vi "batch processor.vi"() -> ()   [LabVIEW 2013]
uses:
  <vilib>/Utility/miscctls.llb/LVPointTypeDef.ctl
  <userlib>/Accelerator/User Interface/Controls/Post_Dust_Event.ctl
  <userlib>/Accelerator/User Interface/Controls/File_location.ctl
  <userlib>/Accelerator/User Interface/Controls/Post_Dust_Event_small.ctl
  <userlib>/_OpenG.lib/array/array.llb/Slice 1D Array (DBL)__ogtk.vi
  <userlib>/Accelerator/Sub-Polymorphic/update_dust_event_big.vi
  <userlib>/_OpenG.lib/string/string.llb/Trim Whitespace (String)__ogtk.vi
  <userlib>/Accelerator/Sub-Polymorphic/update_dust_event_small.vi
  <userlib>/_OpenG.lib/array/array.llb/Empty 1D Array (String)__ogtk.vi
  <vilib>/addons/database/_DB Variant To Data/Database Variant To Data.xnode
panel:
  out "All Processing Frequencies":dbl[](array[numeric])
  in  "Live Run?":bool
  out "Last live data":timestamp
  out "Timed out?":bool
  in  "Tab Control":T1(tab)
  out "Small?":bool
  in  "Clear IDL Errors":bool
  out "IDL Errors":errorcluster
  out "Test":bool caption="Test Database in use:"
  out "Production":bool=TRUE caption="Production Database in use:"
  out "Events being processed:":i32
  out "Processing Frequency (Hz):":ext=3.0
  out "Database Update Progress:":u8(slide) scale=0.0..100.0
  out "IDL Code Executing":bool=TRUE
  out "Estimated IDL Progress:":u8(slide) scale=0.0..100.0
  out "standard error":string
  out "standard output":string
  out "Processing Old Data":bool
  out "Estimated processing time":string="0 days, 0 h, 0 m, 0 s."
  out "Estimated end time":timestamp format="%<%X\n%x>T"
  out "Quality":ext format="%.2f"
  out "Charge":ext
  out "Velocity":ext
  out "Time taken by IDL per shot: (s)":dbl=0.25
  out "Shot being processed:":string
  out "Remaining Shots:":string
  out "Output to IDL command line:":string="\"C:\\Program Files\\Exelis\\IDL82\\bin\\bin.x86_64\\idl.exe\" -e  \"idl_batch_processor, 'X:'\""
  out "Estimate time to process":string="0 s."
  out "Estimate stop time":timestamp format="%<%X\n%x>T"
  out "Total Events":i64
  in  "Lower Time Stamp":timestamp
  in  "Upper Time Stamp":timestamp
  in  "Process old data":bool
  in  "Search Times":bool
  in  "Process all errored entries":bool
  in  "stop":bool
  # "Database Update System V2"
  # "You can ALWAYS run the accelerator.\n\nThis will continue to update the Live\nPlot even if it is processing old data."
  # "Error Status:"
  # "ODBC Connection Status:"
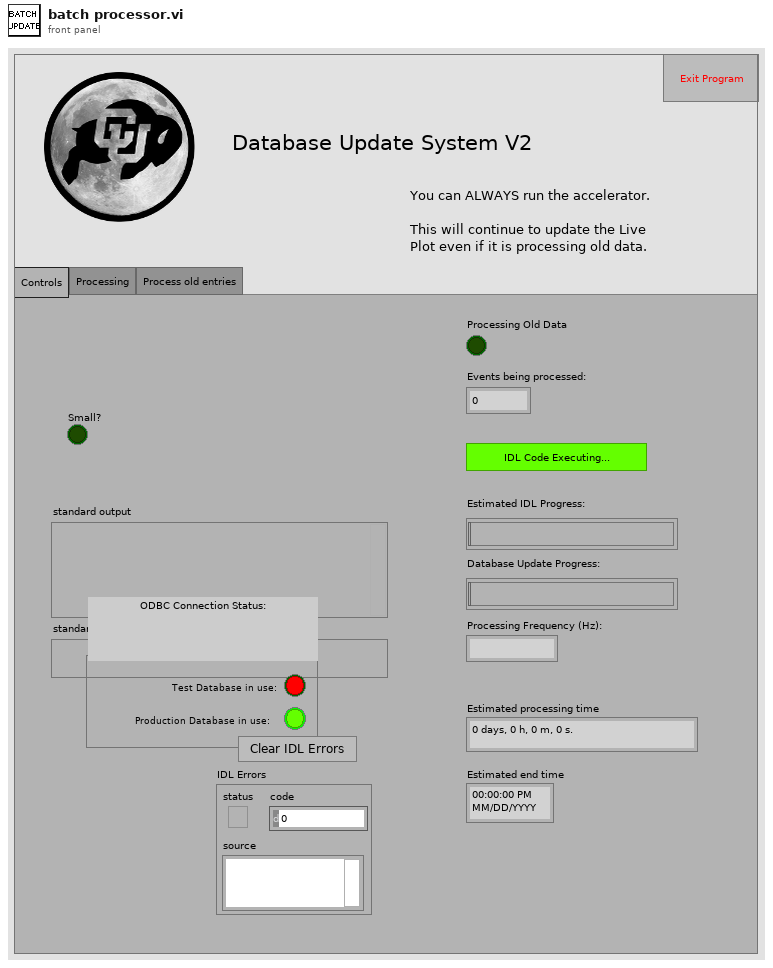
[diagram p1: front panel]
types:
  T1 = enum32{"Controls", "Processing", "Process old entries"}
  T2 = typedef "LVPointTypeDef.ctl" = cluster{"Horizontal":i16, "Vertical":i16}
  T3 = enum8{"Enabled", "Disabled", "Disabled and Grayed Out"}
  T4 = enum16{"open", "replace", "create", "open or create", "replace or create", "replace or create with confirmation"}
  T5 = typedef "Post_Dust_Event.ctl" = cluster{"Dust Event ID":i64, "Integer Timestamp":i64, "Velocity":sgl, "Mass":sgl, "Charge":sgl, "Radius":sgl, "Experiment Settings":dbl, "Pelletron ID":i32, "Estimate Quality":sgl, "File Location":T6, "id_dust_info":dbl, "DCS 1 X":sgl, "DCS 1 Y":sgl, "DCS 2 X":sgl, "DCS 2 Y":sgl}
  T6 = typedef "File_location.ctl" = i8
  T7 = typedef "Post_Dust_Event_small.ctl" = cluster{"Dust Event ID":i64, "Integer Timestamp":i64, "Velocity":sgl, "Mass":sgl, "Charge":sgl, "Radius":sgl, "Needle Voltage (MV)":dbl, "Experiment Settings":dbl, "Estimate Quality":sgl, "File Location":T6, "id_dust_info":dbl}
  T8 = typedef "bp_cluster.ctl" = cluster{"Dust Event ID":i64, "High Voltage":sgl, "Experiment Settings  ID":i64, "File Location":T6, "Dust Density":dbl}
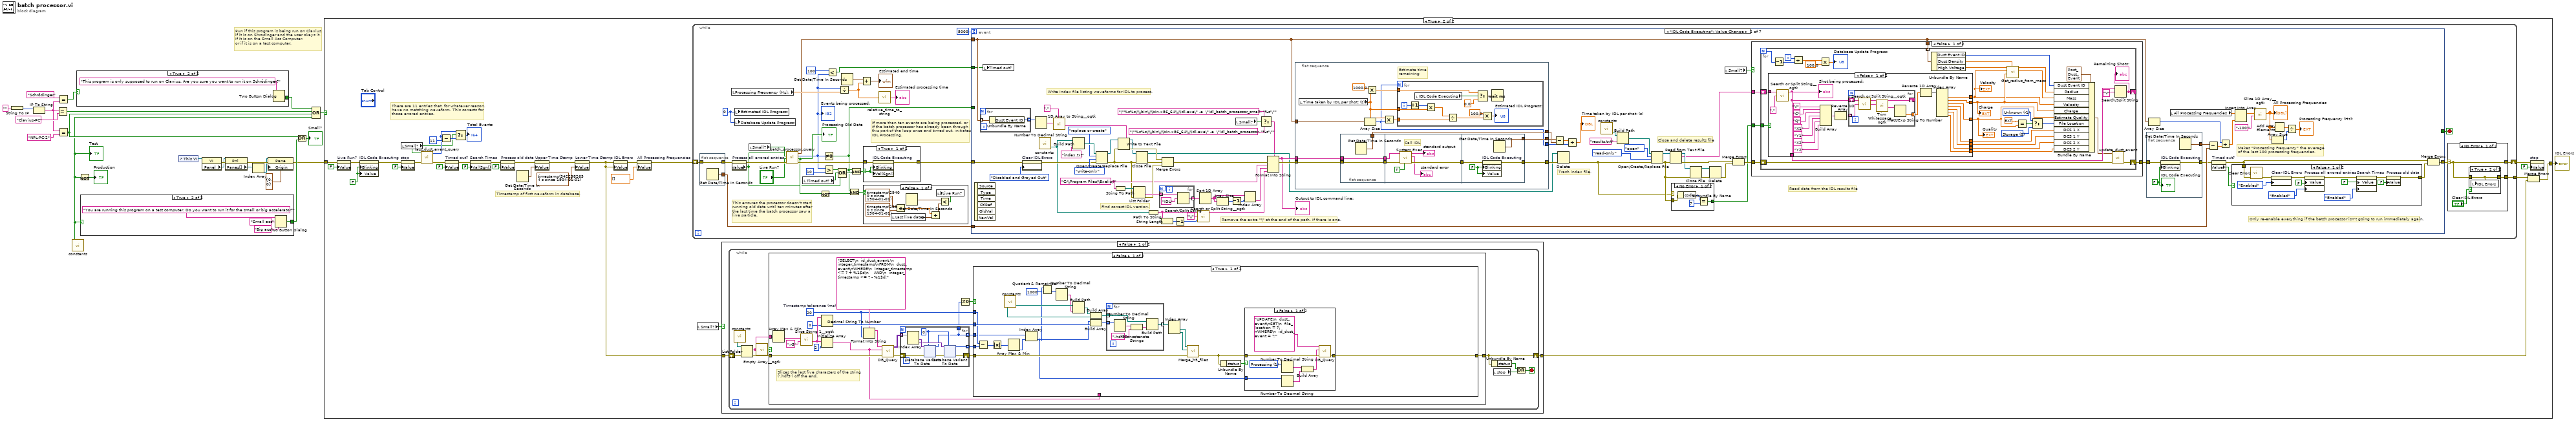
[diagram p0: block diagram]
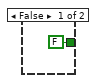
[diagram p2: hidden frame]
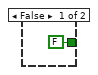
[diagram p3: hidden frame]
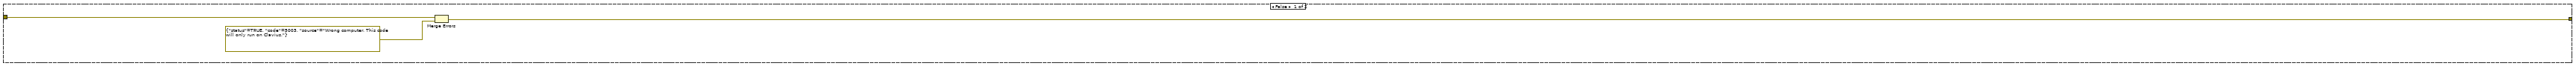
[diagram p4: hidden frame]
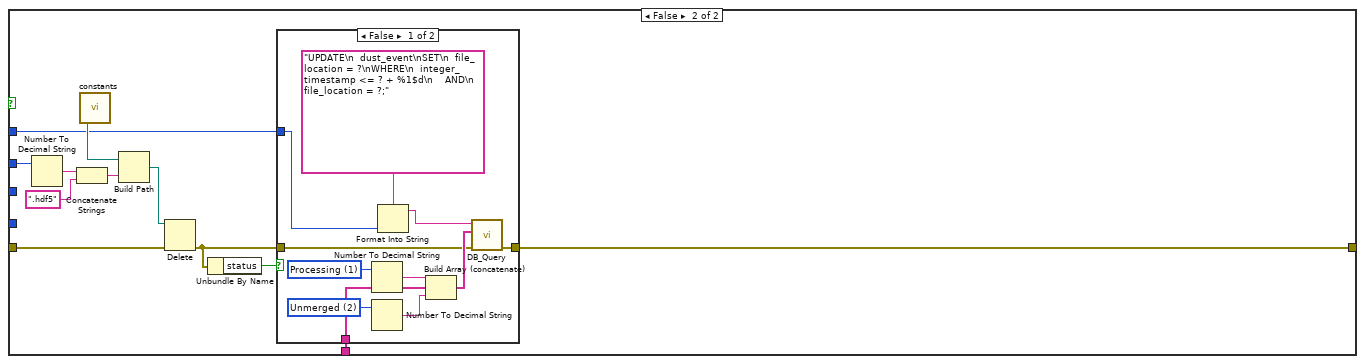
[diagram p6: hidden frame]
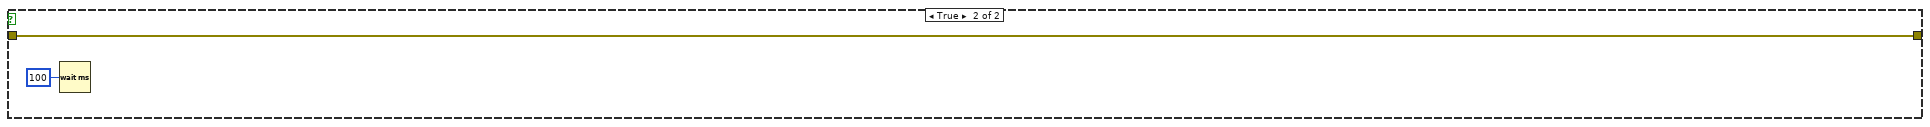
[diagram p8: hidden frame]
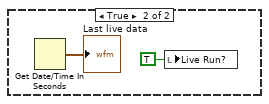
[diagram p10: hidden frame]
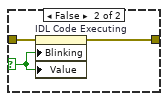
[diagram p11: hidden frame]
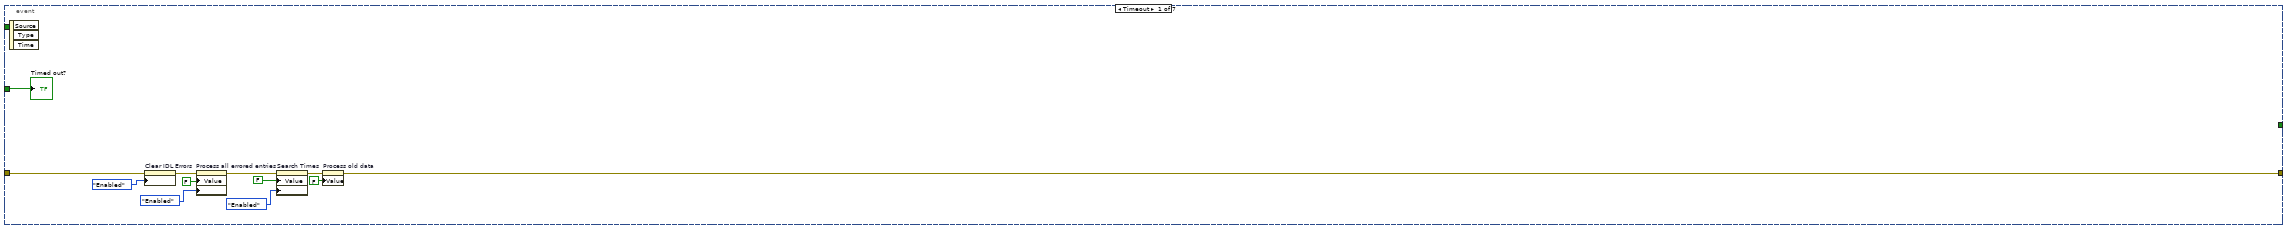
[diagram p12: hidden frame]
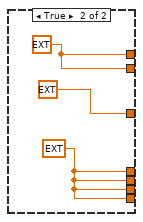
[diagram p13: hidden frame]
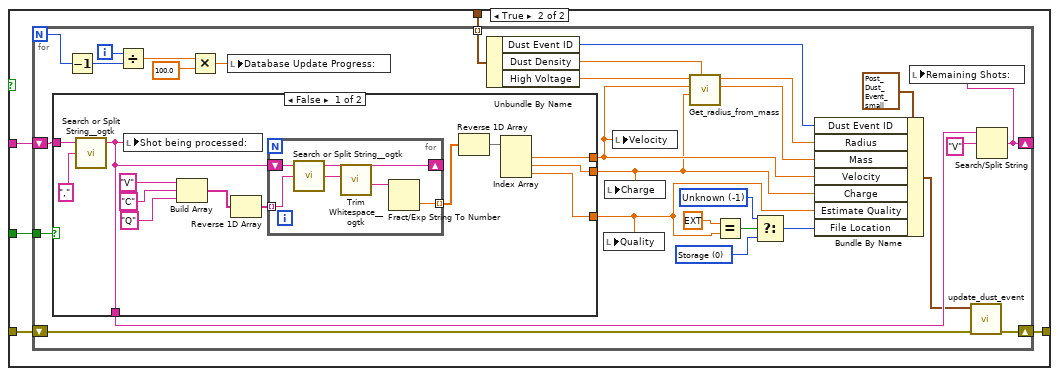
[diagram p14: hidden frame]
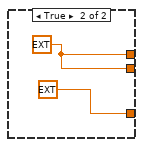
[diagram p15: hidden frame]
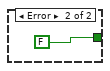
[diagram p17: hidden frame]
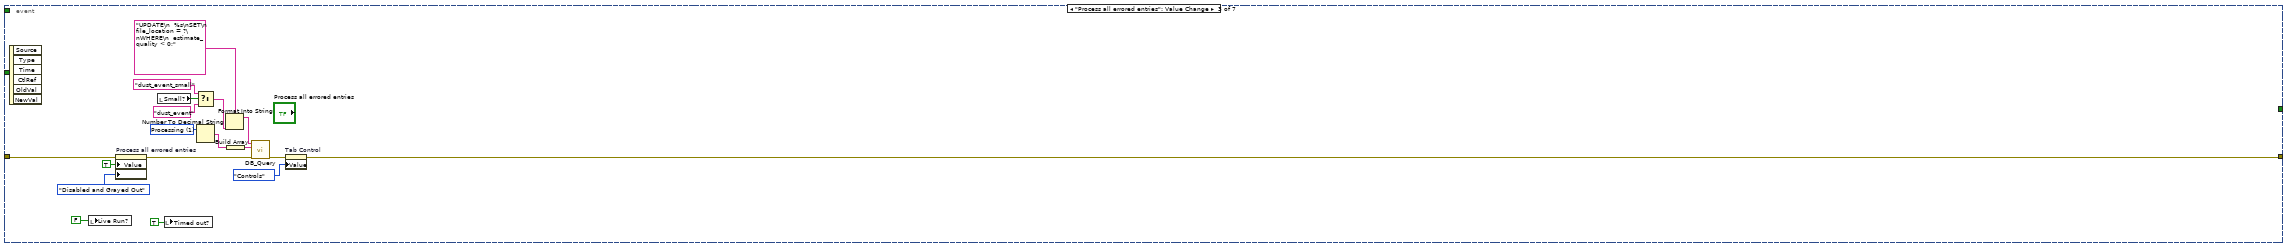
[diagram p18: hidden frame]
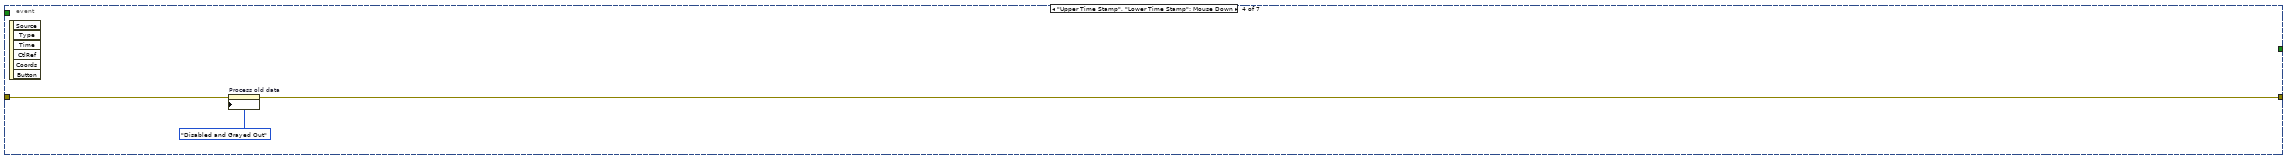
[diagram p19: hidden frame]
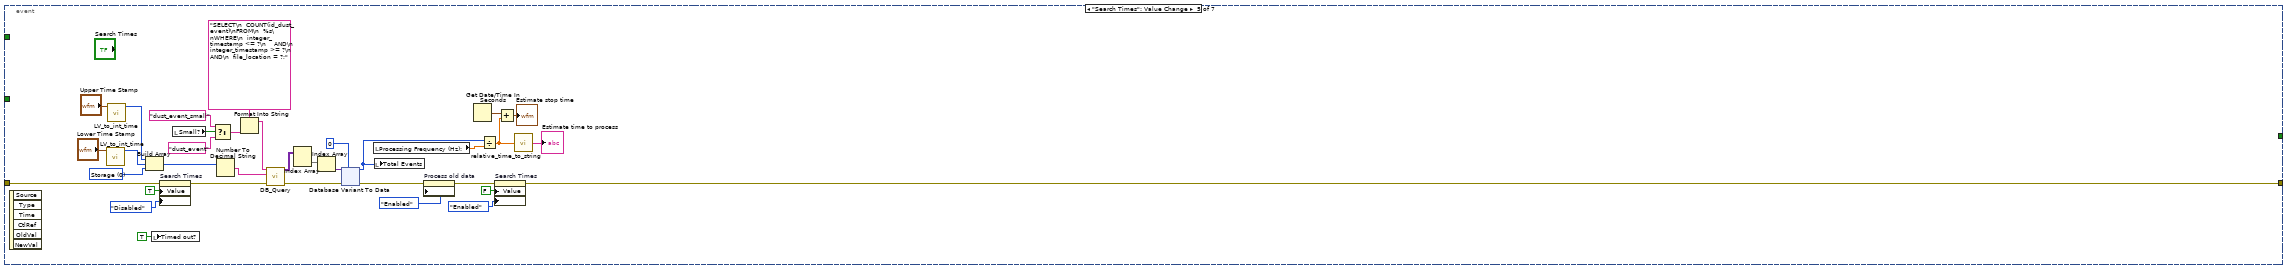
[diagram p20: hidden frame]
diagram:
  # "Run if this program is being run on Clavius,\nif it is on Shrodinger and the user okays it,\nif it is on the Small Acc Computer,\nor if it is on a test computer."
  n1 = String To IP(1:"" ("name")) -> (0:w17:u32)
  n2 = IP To String(2:w17) -> (0:w7:string)  [unwired: 1 in]
  n3 = Equal?(x=w7, y="Clavius-PC") -> (x = y?=w12:bool)
  n4 = Equal?(x="Schrödinger", y=w7) -> (x = y?=w10:bool)
  n5 = Equal?(x=w7, y="NPL-PC-2") -> (x = y?=w5:bool)
  n6 = call <userlib>:"constants.vi"() -> ("Testing"=w1:bool)  [unwired: 3 out]
  "Test" <- w1
  n7 = case shown="True" w10 {
    tunnel: [FALSE ("T button?") w27] -> w11
    frame False {
    }
    frame True {
      n8 = Two Button Dialog(message="This program is only supposed to run on Clavius. Are you sure you want to run it on Schrödinger?") -> (T button?=w27:bool)  [unwired: 2 in]
    }
  }
  n9 = Not(x=w1) -> (.not. x?=→"Production":bool)
  n10 = case shown="True" w1 {
    tunnel: [FALSE ("T button?") w32] -> w4
    frame False {
    }
    frame True {
      n11 = Two Button Dialog(message="You are running this program on a test computer. Do you want to run it for the small or big accelerator?", 1:"Big acc" ("F button name (\"Cancel\")"), 2:"Small acc" ("T button name (\"OK\")")) -> (T button?=w32:bool)
    }
  }
  n12 = control-ref of="This VI"() -> (w24:refnum<vi>)
  n13 = property class="VI"(reference=w24) -> (error out=w23:errorcluster, "Panel"=w22:refnum<vi>)  [unwired: 1 in, 1 out]
  n14 = property class="Pnl"(reference=w22, error in=w23) -> (error out=w21:errorcluster, "Panes[]"=w20:refnum<vi>[])  [unwired: 1 out]
  n15 = Index Array(array=w20) -> (element=w19:refnum<vi>)  [unwired: 1 in]
  n16 = property class="Pane"(reference=w19, error in=w21, "Origin"=T2 {"Horizontal"=0, "Vertical"=0}) -> (error out=w3:errorcluster)  [unwired: 1 out]
  n17 = Or(x=w5, y=w4) -> (x .or. y?=→"Small?":bool)
  n18 = Compound Arithmetic op=OR(w11, w12, w5, w1) -> (w9:bool)
  n19 = case shown="True" w9 {
    tunnel: w3 -> [w35 w41]
    tunnel: [w33 w37] -> w14
    frame False {
      n20 = Merge Errors(w35, errorcluster {"status"=TRUE, "code"=5003, "source"="Wrong computer. This code will only run on Clavius."} ("error IO")) -> (w33:errorcluster)
    }
    frame True {
      w67 = FALSE ("IDL Code Executing")
      # "There are 11 entries that, for whatever reason,\nhave no matching waveform. This corrects for\nthose errored entries."
      # "Timestamp of first waveform in database."
      n21 = property on="Live Run?" class="Bool (strict)"(error in=w41, "Value"=FALSE ("Live Run?")) -> (error out=w50:errorcluster)  [unwired: 1 in, 1 out]
      n22 = property on="IDL Code Executing" class="Bool (strict)"(error in=w50, "Blinking"=w67, "Value"=w67) -> (error out=w64:errorcluster)  [unwired: 1 in, 1 out]
      n23 = property on="stop" class="Bool (strict)"(error in=w64, "Value"=FALSE ("stop")) -> (error out=w54:errorcluster)  [unwired: 1 in, 1 out]
      n24 = local read "Small?"() -> (w42:bool)
      n25 = call <userlib>:"last_dust_event_query.vi"("error in (no error)"=w54, "Small?"=w42) -> ("error out"=w53:errorcluster, "id_dust_event"=w43:i64)  [unwired: 8 in]
      n26 = Subtract(x=w43, y=i64 11) -> (x-y=w44:i64)
      n27 = property on="Timed out?" class="Bool (strict)"(error in=w53, "Value"=FALSE ("stop")) -> (error out=w58:errorcluster)  [unwired: 1 in, 1 out]
      n28 = Select(t=w43, s=w42, f=w44) -> (s? t:f=→"Total Events":i64)
      n29 = property on="Search Times" class="Bool (strict)"(error in=w58, "Val(Sgnl)"=FALSE ("Search Times")) -> (error out=w56:errorcluster)  [unwired: 1 in, 1 out]
      n30 = property on="Process old data" class="Bool (strict)"(error in=w56, "Value"=FALSE ("Process old data")) -> (error out=w51:errorcluster)  [unwired: 1 in, 1 out]
      n31 = Get Date/Time In Seconds() -> (seconds since 1Jan1904=w62:timestamp)
      n32 = property on="Upper Time Stamp" class="AbsTime (strict)"(error in=w51, "Value"=w62) -> (error out=w61:errorcluster)  [unwired: 1 in, 1 out]
      n33 = property on="Lower Time Stamp" class="AbsTime (strict)"(error in=w61, "Value"=timestamp(3422982654.564 s since 1904-01-01) ("Upper Time Stamp")) -> (error out=w40:errorcluster)  [unwired: 1 in, 1 out]
      n34 = property on="IDL Errors" class="Clust (strict)"(error in=w40, "Value"=w40) -> (error out=w48:errorcluster)  [unwired: 1 in, 1 out]
      n35 = property on="All Processing Frequencies" class="Arr (strict)"(error in=w48, "Value"=dbl[] [] ("All Processing Frequencies")) -> (error out=w46:errorcluster)  [unwired: 1 in, 1 out]
      n36 = while {
        shift-right: [w265] -> w65
        shift-left: w46 -> [w254]
        tunnel: [w264] -> w38
        stop <- w260 stop-if-true
        w268 = u8 0 ("Database Update Progress")
        # "This ensures the processor doesn't start\nrunning old data until ten minutes after\nthe last time the batch processor saw a\nlive particle."
        # "If more than ten events are being processed, or\nif the batch processor has already been through\nthis part of the loop once and timed out, initiates\nIDL Processing."
        n37 = flat-sequence {
          tunnel: [w279] -> w255
          tunnel: w254 -> [w279]
          tunnel: [w278] -> w253
          frame #0 {
            n38 = Get Date/Time In Seconds() -> (seconds since 1Jan1904=w278:timestamp)
          }
        }
        n39 = local read "Processing Frequency (Hz):"() -> (w245:ext)
        n40 = property on="Process all errored entries" class="Bool (strict)"(error in=w255) -> (error out=w259:errorcluster, "Value"=w241:bool)  [unwired: 1 in, 1 out]
        n41 = local write "Estimated IDL Progress:"(w268) -> ()
        n42 = local write "Database Update Progress:"(w268) -> ()
        n43 = local read "Small?"() -> (w252:bool)
        n44 = call <userlib>:"batch_processor_query.vi"("error in (no error)"=w259, "Live Run?"="Live Run?", "Small?"=w252, "Update Error files?"=w241) -> ("error out"=w262:errorcluster, "Old Processing"=w248:bool, "Total Events"=w237:i32, "BP Array"=w236:T8[])  [unwired: 4 in]
        "Events being processed:" <- w237
        "Processing Old Data" <- w248
        n45 = local read "Timed out?"() -> (w256:bool)
        n46 = Not(x=w248) -> (.not. x?=w247:bool)
        n47 = Not Equal To 0?(x=w237) -> (x != 0?=w240:bool)
        n48 = Greater?(x=w237, y=10) -> (0:w258:bool)
        n49 = Less?(x=100 ("length"), y=w237) -> (x < y?=w238:bool)
        n50 = Compound Arithmetic op=OR(w258, w256, w241) -> (w251:bool)
        n51 = Divide(x=w237, y=w245) -> (x/y=w243:ext)
        n52 = Get Date/Time In Seconds() -> (seconds since 1Jan1904=w246:timestamp)
        n53 = And(x=w240, y=w247) -> (x .and. y?=w249:bool)
        n54 = And(x=w240, y=w251) -> (x .and. y?=w257:bool)
        n55 = Add(x=w246, y=w243) -> (x+y=→"Estimated end time":timestamp)
        n56 = case shown="True" w257 {
          selector: w257 -> [w280 w283]
          tunnel: w262 -> [w282 w285]
          tunnel: [w281 w284] -> w261
          frame True {
            n57 = property on="IDL Code Executing" class="Bool (strict)"(error in=w282, "Blinking"=w280, "Val(Sgnl)"=w280) -> (error out=w281:errorcluster)  [unwired: 1 in, 1 out]
          }
          frame False {
            n58 = property on="IDL Code Executing" class="Bool (strict)"(error in=w285, "Blinking"=w283, "Value"=w283) -> (error out=w284:errorcluster)  [unwired: 1 in, 1 out]
          }
        }
        n59 = case shown="False" w249 {
          frame False {
            n60 = local read "Last live data"() -> (w275:timestamp)
            n61 = Subtract(x=timestamp(29400 s since 1904-01-01) ("Last live data"), y=timestamp(28800 s since 1904-01-01) ("Last live data")) -> (x-y=w274:dbl)
            n62 = Get Date/Time In Seconds() -> (seconds since 1Jan1904=w270:timestamp)
            n63 = Add(x=w274, y=w275) -> (x+y=w269:timestamp)
            n64 = Less?(x=w270, y=w269) -> (x < y?=w271:bool)
            n65 = local write "Live Run?"(w271) -> ()
          }
          frame True {
            n66 = Get Date/Time In Seconds() -> (seconds since 1Jan1904=→"Last live data":timestamp)
            n67 = local write "Live Run?"(TRUE ("Live Run?")) -> ()
          }
        }
        n68 = call <userlib>:"relative_time_to_string.vi"("Seconds"=w243) -> ("String time"=→"Estimated processing time":string)
        n69 = event shown="[1] \"IDL Code Executing\": Value Change" {
          selector: _ -> [_ _ _ _ _ _ _]
          dyn-events: _ -> [_ _ _ _ _ _ _]
          timeout: 5000 -> [_ _ _ _ _ _ _]
          tunnel: w261 -> [w288 w325 w582 w588 w604 w663 w683]
          tunnel: w236 -> [_ w315 _ _ _ _ _]
          tunnel: [w287 w322 w586 w587 w612 w677 w683] -> w266
          tunnel: [_ _ _ _ _ _ "stop"] -> w260
          tunnel: w253 -> [_ w316 _ _ _ _ _]
          tunnel: w240 -> [w286 _ _ _ _ _ _]
          tunnel: w238 -> [_ w313 _ _ _ _ _]
          event Timeout {
            n70 = event-data() -> ()  [unwired: 1 in, 3 out]
            n71 = property on="Clear IDL Errors" class="Bool"(error in=w288, "DisabledEnum"=T3."Enabled" ("Disabled")) -> (error out=w294:errorcluster)  [unwired: 1 in, 1 out]
            n72 = property on="Process all errored entries" class="Bool (strict)"(error in=w294, "Value"=FALSE ("Process old errored entries"), "DisabledEnum"=T3."Enabled" ("Disabled")) -> (error out=w295:errorcluster)  [unwired: 1 in, 1 out]
            n73 = property on="Search Times" class="Bool (strict)"(error in=w295, "Value"=FALSE ("Process old data"), "DisabledEnum"=T3."Enabled" ("Disabled")) -> (error out=w296:errorcluster)  [unwired: 1 in, 1 out]
            n74 = property on="Process old data" class="Bool (strict)"(error in=w296, "Value"=FALSE ("Process old data")) -> (error out=w287:errorcluster)  [unwired: 1 in, 1 out]
            "Timed out?" <- w286
          }
          event "IDL Code Executing": Value Change {
            w347 = "C:\\Program Files\\Exelis\\"
            # "Makes \"Processing Frequency\" the average\nof the last 100 processing frequencies."
            # "Only re-enable everything if the batch processor isn't going to run immediately again."
            # "Close and delete results file"
            # "Read data from the IDL results file"
            # "Trash index file."
            # "Remove the extra \"\\\" at the end of the path, if there is one."
            # "Find correct IDL version."
            # "Write index file listing waveforms for IDL to process."
            n75 = event-data() -> ()  [unwired: 1 in, 6 out]
            n76 = for {
              tunnel: w315 -> [w517] mode=indexing
              tunnel: [w516] -> w344 mode=indexing
              n77 = Unbundle By Name(w517) -> ("Dust Event ID"=w516:i64)
            }
            n78 = local write "Timed out?"(w313) -> ()
            n79 = property on="Clear IDL Errors" class="Bool"(error in=w325, "DisabledEnum"=T3."Disabled and Grayed Out" ("Disabled")) -> (error out=w301:errorcluster)  [unwired: 1 in, 1 out]
            n80 = Number To Decimal String(number=w344) -> (decimal integer string=w340:string[])  [unwired: 1 in]
            n81 = call <userlib>:"constants.vi"() -> ("Processed HDF5 filepath"=w300:path)  [unwired: 3 out]
            n82 = call <userlib>:"1D Array to String__ogtk.vi"("delimiter (Tab)"=",", "Array of Strings"=w340) -> ("delimited string"=w338:string)  [unwired: 9 in]
            n83 = Build Path(base path=w300, name or relative path="index.txt") -> (appended path=w378:path)
            n84 = Open/Create/Replace File(file path (use dialog)=w378, error in=w301, operation (0:open)=T4."replace or create", access (0:read/write)=enum16{"read/write", "read-only", "write-only"}."write-only") -> (refnum out=w341:refnum<file>, error out=w337:errorcluster)  [unwired: 2 in, 1 out]
            n85 = String To Path(string=w347) -> (path=w359:path)
            n86 = Write to Text File(file (use dialog)=w341, text=w338, error in=w337) -> (refnum out=w342:refnum<file>, error out=w343:errorcluster)  [unwired: 1 in, 1 out]
            n87 = List Folder(path=w359, error in=w337) -> (folder names=w358:string[], error out=w348:errorcluster)  [unwired: 2 in, 2 out]
            n88 = Close File(refnum=w342, error in=w337) -> (path=w330:path, error out=w377:errorcluster)
            n89 = Path To String(path=w300) -> (string=w350:string)
            n90 = for {
              tunnel: w358 -> [w519] mode=indexing
              tunnel: [w518] -> w356 mode=indexing
              n91 = Search/Split String(string=w519, search string/char (-)="IDL" ("Element Data")) -> (match + rest of string=w518:string)  [unwired: 1 in, 2 out]
            }
            n92 = String Length(string=w350) -> (length=w352:i32)
            n93 = Merge Errors(w343, w377, w348) -> (w370:errorcluster)
            n94 = Decrement(x=w352) -> (x-1=w351:i32)
            n95 = call <userlib>:"Search or Split String__ogtk.vi"("offset (0)"=w351, "search string/char (-)"="\\", "string"=w350) -> ("substring before match"=w345:string)  [unwired: 2 out]
            n96 = Sort 1D Array(array=w356) -> (sorted array=w357:string[])
            n97 = Array Size(array=w357) -> (size(s)=w355:i32)
            n98 = Decrement(x=w355) -> (x-1=w354:i32)
            n99 = local read "Small?"() -> (w320:bool)
            n100 = Index Array(array=w357, index=w354) -> (element=w346:string)
            n101 = Select(t="\"%s%s\\\\bin\\\\bin.x86_64\\\\idl.exe\" -e  \"idl_batch_processor_small, '%s'\"" ("format string"), s=w320, f="\"%s%s\\\\bin\\\\bin.x86_64\\\\idl.exe\" -e  \"idl_batch_processor, '%s'\"" ("format string")) -> (s? t:f=w317:string)
            n102 = Format Into String(format string=w317, error in=w370, w347, w346, w345) -> (resulting string=w353:string, error out=w371:errorcluster)  [unwired: 1 in]
            "Output to IDL command line:" <- w353
            n103 = flat-sequence {
              tunnel: w371 -> [w542]
              tunnel: w353 -> [w543]
              tunnel: [w541] -> w331
              tunnel: [w534] -> w336
              tunnel: [w533] -> w335
              tunnel: [w531] -> w333
              tunnel: w315 -> [w530]
              frame #0 {
                # "Estimate time \nremaining"
                n104 = local read "Time taken by IDL per shot: (s)"() -> (w532:dbl)
                n105 = flat-sequence {
                  tunnel: w542 -> [w557]
                  tunnel: w543 -> [w558]
                  tunnel: [w558] -> w539
                  tunnel: [w557] -> w538
                  tunnel: [w556] -> w533
                  tunnel: [w562] -> w540
                  tunnel: w539 -> [w564]
                  tunnel: w538 -> [w563]
                  tunnel: [w568] -> w534
                  tunnel: [w565] -> w541
                  tunnel: w540 -> [w566]
                  frame #0 {
                    n106 = Get Date/Time In Seconds() -> (seconds since 1Jan1904=w556:timestamp)
                  }
                  frame #1 {
                    # "Call IDL"
                    n107 = call <vilib>:"System Exec.vi"("run minimized? (F)"=TRUE, "error in (no error)"=w563, "command line"=w564) -> ("error out"=w562:errorcluster, "standard error"=→"standard error":string, "standard output"=→"standard output":string)  [unwired: 5 in, 1 out]
                  }
                  frame #2 {
                    w567 = FALSE ("IDL Code Executing")
                    n108 = property on="IDL Code Executing" class="Bool (strict)"(error in=w566, "Blinking"=w567, "Value"=w567) -> (error out=w565:errorcluster)  [unwired: 1 in, 1 out]
                    n109 = Get Date/Time In Seconds() -> (seconds since 1Jan1904=w568:timestamp)
                  }
                }
                n110 = Array Size(array=w530) -> (size(s)=w531:i32)
                n111 = Multiply(x=sgl 1000.0 ("y"), y=w532) -> (x*y=w536:dbl)
                n112 = Multiply(x=w532, y=w531) -> (x*y=w535:dbl)
                n113 = for {
                  N: w531 -> [_]
                  tunnel: w535 -> [w551]
                  tunnel: w532 -> [w554]
                  tunnel: w536 -> [w545]
                  i -> [w555]
                  n114 = Increment(x=w555) -> (x+1=w553:i32)
                  n115 = local read "IDL Code Executing"() -> (w547:bool)
                  n116 = Multiply(x=w553, y=w554) -> (x*y=w552:dbl)
                  n117 = Divide(x=w552, y=w551) -> (x/y=w550:dbl)
                  n118 = Select(t=w545, s=w547, f=0.0) -> (s? t:f=w546:dbl)
                  n119 = Multiply(x=sgl 100.0, y=w550) -> (x*y=→"Estimated IDL Progress:":dbl)
                  n120 = Wait (ms)(milliseconds to wait=w546) -> ()  [unwired: 1 out]
                }
              }
            }
            n121 = Subtract(x=w336, y=w335) -> (x-y=w334:dbl)
            n122 = Delete(path (use dialog)=w330, error in=w331) -> (error out=w332:errorcluster)  [unwired: 3 in, 2 out]
            n123 = Divide(x=w334, y=w333) -> (x/y=→"Time taken by IDL per shot: (s)":dbl)
            n124 = call <userlib>:"constants.vi"() -> ("Processed HDF5 filepath"=w299:path)  [unwired: 3 out]
            n125 = Build Path(base path=w299, name or relative path="results.txt") -> (appended path=w375:path)
            n126 = Open/Create/Replace File(file path (use dialog)=w375, error in=w332, operation (0:open)=T4."open", access (0:read/write)=enum16{"read/write", "read-only", "write-only"}."read-only") -> (refnum out=w374:refnum<file>, error out=w361:errorcluster)  [unwired: 2 in, 1 out]
            n127 = Read from Text File(file (use dialog)=w374, error in=w361) -> (refnum out=w365:refnum<file>, text=w364:string, error out=w373:errorcluster)  [unwired: 2 in, 1 out]
            n128 = case shown="No Error" w332 {
              tunnel: w361 -> [w524 _]
              tunnel: [w521 FALSE] -> w360
              frame No Error {
                n129 = Unbundle By Name(w524) -> ("code"=w523:i32)
                n130 = Equal?(x=w523, y=7) -> (x = y?=w521:bool)
              }
              frame Error {
              }
            }
            n131 = Close File(refnum=w365, error in=w361) -> (path=w329:path, error out=w327:errorcluster)
            n132 = Delete(path (use dialog)=w329, error in=w327) -> (error out=w326:errorcluster)  [unwired: 3 in, 2 out]
            n133 = local read "Small?"() -> (w298:bool)
            n134 = Merge Errors(w373, w326) -> (w372:errorcluster)
            n135 = case shown="False" w298 {
              tunnel: w372 -> [w384 w452]
              tunnel: w364 -> [w383 w451]
              tunnel: w360 -> [w382 w450]
              tunnel: [w381 w449] -> w328
              tunnel: w315 -> [w380 w448]
              frame False {
                n136 = for {
                  N -> [w409]
                  shift-right: [w390] -> w381
                  shift-left: w384 -> [w391]
                  tunnel: w380 -> [w417] mode=indexing
                  shift-right: [w385] -> _
                  shift-left: w383 -> [w414]
                  tunnel: w382 -> [w405]
                  i -> [w413]
                  w396 = T6 -1 items=["Unknown"=-1, "Storage"=0, "Processing"=1, "Unmerged"=2] ("File Location")
                  w397 = T6 0 items=["Unknown"=-1, "Storage"=0, "Processing"=1, "Unmerged"=2] ("File Location")
                  n137 = case shown="False" w405 {
                    tunnel: [w422 ext 0.0] -> w399
                    tunnel: [w424 w445] -> w401
                    tunnel: [w423 w445] -> w402
                    tunnel: w414 -> [w438 _]
                    tunnel: [w427 _] -> w407
                    tunnel: [w421 w446] -> w389
                    tunnel: [w420 w446] -> w388
                    tunnel: [w419 w446] -> w387
                    tunnel: [w418 w446] -> w386
                    frame False {
                      n138 = call <userlib>:"Search or Split String__ogtk.vi"("search string/char (-)"=",", "string"=w438) -> ("substring before match"=w427:string)  [unwired: 1 in, 2 out]
                      "Shot being processed:" <- w427
                      n139 = Build Array("V" ("search string/char (-)"), "C" ("search string/char (-)"), "Q" ("search string/char (-)"), "X1" ("search string/char (-)"), "Y1" ("search string/char (-)"), "X2" ("search string/char (-)"), "Y2" ("search string/char (-)")) -> (w429:string[])
                      n140 = Reverse 1D Array(array=w429) -> (reversed array=w428:string[])
                      n141 = for {
                        tunnel: w428 -> [w440] mode=indexing
                        shift-right: [w441] -> _
                        shift-left: w427 -> [w442]
                        tunnel: [w439] -> w426 mode=indexing
                        n142 = call <userlib>:"Search or Split String__ogtk.vi"("search string/char (-)"=w440, "string"=w442) -> ("substring after match"=w443:string, "substring before match"=w441:string)  [unwired: 1 in, 1 out]
                        n143 = call-poly <userlib>:"Trim Whitespace__ogtk.vi"("String in"=w443) -> ("String out"=w444:string)  [unwired: 6 in]
                        n144 = Fract/Exp String To Number(string=w444) -> (number=w439:dbl)  [unwired: 3 in, 1 out]
                      }
                      n145 = Reverse 1D Array(array=w426) -> (reversed array=w425:dbl[])
                      n146 = Index Array(array=w425) -> (element #1=w424:dbl, element #2=w423:dbl, element #3=w422:dbl, element #4=w421:dbl, element #5=w420:dbl, element #6=w419:dbl, element #7=w418:dbl)  [unwired: 7 in]
                    }
                    frame True {
                      w446 = ext -99.0
                      w445 = ext -5.0
                    }
                  }
                  "Quality" <- w399
                  "Charge" <- w402
                  "Velocity" <- w401
                  n147 = Decrement(x=w409) -> (x-1=w408:i32)
                  n148 = Divide(x=w413, y=w408) -> (x/y=w412:dbl)
                  n149 = Multiply(x=w412, y=100.0) -> (x*y=→"Database Update Progress:":dbl)
                  n150 = Unbundle By Name(w417) -> ("Dust Event ID"=w394:i64, "Dust Density"=w403:dbl, "High Voltage"=w404:sgl)
                  n151 = call <userlib>:"Get_radius_from_mass.vi"("Density (g/cc)"=w403, "Charge"=w402, "Velocity"=w401, "High Voltage (MV)"=w404) -> ("Mass"=w415:ext, "Radius"=w400:dbl)  [unwired: 6 in]
                  n152 = Equal?(x=ext -4.0, y=w399) -> (x = y?=w395:bool)
                  n153 = Select(t=w396, s=w395, f=w397) -> (s? t:f=w393:T6)
                  n154 = Bundle By Name(cluster=T5 {"Dust Event ID"=0, "Integer Timestamp"=0, "Velocity"=0.0, "Mass"=0.0, "Charge"=0.0, "Radius"=0.0, "Experiment Settings"=0.0, "Pelletron ID"=0, "Estimate Quality"=0.0, "File Location"=0, "id_dust_info"=0.0, "DCS 1 X"=0.0, "DCS 1 Y"=0.0, "DCS 2 X"=0.0, "DCS 2 Y"=0.0} ("Cluster"), "Dust Event ID"=w394, "Radius"=w400, "Mass"=w415, "Velocity"=w401, "Charge"=w402, "Estimate Quality"=w399, "File Location"=w393, "DCS 1 X"=w389, "DCS 1 Y"=w388, "DCS 2 X"=w387, "DCS 2 Y"=w386) -> (w392:T5)
                  n155 = call-poly <userlib>:"update_dust_event.vi"("error in (no error)"=w391, "Cluster"=w392) -> ("error out"=w390:errorcluster)  [unwired: 9 in]
                  n156 = Search/Split String(string=w407, search string/char (-)="V") -> (match + rest of string=w385:string)  [unwired: 1 in, 2 out]
                  "Remaining Shots:" <- w385
                }
              }
              frame True {
                n157 = for {
                  N -> [w474]
                  shift-right: [w458] -> w449
                  shift-left: w452 -> [w459]
                  tunnel: w448 -> [w481] mode=indexing
                  shift-right: [w453] -> _
                  shift-left: w451 -> [w478]
                  tunnel: w450 -> [w470]
                  i -> [w477]
                  w464 = T6 -1 items=["Unknown"=-1, "Storage"=0, "Processing"=1, "Unmerged"=2] ("File Location")
                  w465 = T6 0 items=["Unknown"=-1, "Storage"=0, "Processing"=1, "Unmerged"=2] ("File Location")
                  n158 = case shown="False" w470 {
                    tunnel: [w483 ext 0.0] -> w455
                    tunnel: [w485 w501] -> w457
                    tunnel: [w484 w501] -> w456
                    tunnel: w478 -> [w494 _]
                    tunnel: [w482 _] -> w472
                    frame False {
                      n159 = call <userlib>:"Search or Split String__ogtk.vi"("search string/char (-)"=",", "string"=w494) -> ("substring before match"=w482:string)  [unwired: 1 in, 2 out]
                      n160 = local write "Shot being processed:"(w482) -> ()
                      n161 = Build Array("V" ("search string/char (-)"), "C" ("search string/char (-)"), "Q" ("search string/char (-)")) -> (w489:string[])
                      n162 = Reverse 1D Array(array=w489) -> (reversed array=w488:string[])
                      n163 = for {
                        tunnel: w488 -> [w496] mode=indexing
                        shift-right: [w497] -> _
                        shift-left: w482 -> [w498]
                        tunnel: [w495] -> w487 mode=indexing
                        n164 = call <userlib>:"Search or Split String__ogtk.vi"("search string/char (-)"=w496, "string"=w498) -> ("substring after match"=w499:string, "substring before match"=w497:string)  [unwired: 1 in, 1 out]
                        n165 = call-poly <userlib>:"Trim Whitespace__ogtk.vi"("String in"=w499) -> ("String out"=w500:string)  [unwired: 6 in]
                        n166 = Fract/Exp String To Number(string=w500) -> (number=w495:dbl)  [unwired: 3 in, 1 out]
                      }
                      n167 = Reverse 1D Array(array=w487) -> (reversed array=w486:dbl[])
                      n168 = Index Array(array=w486) -> (element #1=w485:dbl, element #2=w484:dbl, element #3=w483:dbl)  [unwired: 3 in]
                    }
                    frame True {
                      w501 = ext -5.0
                    }
                  }
                  n169 = Decrement(x=w474) -> (x-1=w473:i32)
                  n170 = Divide(x=w477, y=w473) -> (x/y=w476:dbl)
                  n171 = Multiply(x=w476, y=100.0) -> (x*y=w454:dbl)
                  n172 = local write "Database Update Progress:"(w454) -> ()
                  n173 = Unbundle By Name(w481) -> ("Dust Event ID"=w462:i64, "Dust Density"=w468:dbl, "High Voltage"=w469:sgl)
                  n174 = local write "Quality"(w455) -> ()
                  n175 = local write "Charge"(w456) -> ()
                  n176 = local write "Velocity"(w457) -> ()
                  n177 = call <userlib>:"Get_radius_from_mass.vi"("Density (g/cc)"=w468, "Charge"=w456, "Velocity"=w457, "High Voltage (MV)"=w469) -> ("Mass"=w479:ext, "Radius"=w467:dbl)  [unwired: 6 in]
                  n178 = Equal?(x=ext -4.0, y=w455) -> (x = y?=w463:bool)
                  n179 = Select(t=w464, s=w463, f=w465) -> (s? t:f=w461:T6)
                  n180 = Bundle By Name(cluster=T7 {"Dust Event ID"=0, "Integer Timestamp"=0, "Velocity"=0.0, "Mass"=0.0, "Charge"=0.0, "Radius"=0.0, "Needle Voltage (MV)"=0.0, "Experiment Settings"=0.0, "Estimate Quality"=0.0, "File Location"=0, "id_dust_info"=0.0} ("Cluster"), "Dust Event ID"=w462, "Radius"=w467, "Mass"=w479, "Velocity"=w457, "Charge"=w456, "Estimate Quality"=w455, "File Location"=w461) -> (w460:T7)
                  n181 = call-poly <userlib>:"update_dust_event.vi"("error in (no error)"=w459, "Cluster"=w460) -> ("error out"=w458:errorcluster)  [unwired: 9 in]
                  n182 = Search/Split String(string=w472, search string/char (-)="V") -> (match + rest of string=w453:string)  [unwired: 1 in, 2 out]
                  n183 = local write "Remaining Shots:"(w453) -> ()
                }
              }
            }
            n184 = flat-sequence {
              tunnel: w328 -> [w528]
              tunnel: [w527] -> w312
              tunnel: [w529] -> w362
              frame #0 {
                w526 = FALSE ("IDL Code Executing")
                n185 = property on="IDL Code Executing" class="Bool (strict)"(error in=w528, "Blinking"=w526) -> (error out=w527:errorcluster)  [unwired: 1 in, 1 out]
                n186 = Get Date/Time In Seconds() -> (seconds since 1Jan1904=w529:timestamp)
                "IDL Code Executing" <- w526
              }
            }
            n187 = Array Size(array=w315) -> (size(s)=w314:i32)
            n188 = local read "All Processing Frequencies"() -> (w308:dbl[])
            n189 = Subtract(x=w362, y=w316) -> (x-y=w363:dbl)
            n190 = property on="Timed out?" class="Bool (strict)"(error in=w312) -> (error out=w311:errorcluster, "Value"=w310:bool)  [unwired: 1 in, 1 out]
            n191 = Divide(x=w314, y=w363) -> (x/y=w309:dbl)
            n192 = case shown="False" w310 {
              tunnel: w311 -> [w514 w515]
              tunnel: [w503 w515] -> w321
              frame False {
                n193 = call <vilib>:"Clear Errors.vi"("error in (no error)"=w514) -> ("error out"=w513:errorcluster)  [unwired: 6 in]
                n194 = property on="Clear IDL Errors" class="Bool"(error in=w513, "DisabledEnum"=T3."Enabled" ("Disabled")) -> (error out=w511:errorcluster)  [unwired: 1 in, 1 out]
                n195 = property on="Process all errored entries" class="Bool (strict)"(error in=w511, "Value"=FALSE ("Process old errored entries"), "DisabledEnum"=T3."Enabled" ("Disabled")) -> (error out=w508:errorcluster)  [unwired: 1 in, 1 out]
                n196 = property on="Search Times" class="Bool (strict)"(error in=w508, "Value"=FALSE ("Process old data"), "DisabledEnum"=T3."Enabled" ("Disabled")) -> (error out=w504:errorcluster)  [unwired: 1 in, 1 out]
                n197 = property on="Process old data" class="Bool (strict)"(error in=w504, "Value"=FALSE ("Process old data")) -> (error out=w503:errorcluster)  [unwired: 1 in, 1 out]
              }
              frame True {
              }
            }
            n198 = Insert Into Array(array=w308, new element=w309) -> (w307:dbl[])  [unwired: 1 in]
            n199 = call-poly <userlib>:"Slice 1D Array__ogtk.vi"("slice"="-100:", "array"=w307) -> ("subarray (array[i:j])"=w303:dbl[])  [unwired: 5 in]
            "All Processing Frequencies" <- w303
            n200 = Array Size(array=w303) -> (size(s)=w305:i32)
            n201 = Add Array Elements(numeric array=w303) -> (sum=w306:dbl)
            n202 = Divide(x=w306, y=w305) -> (x/y=→"Processing Frequency (Hz):":dbl)
            n203 = Merge Errors(w311, w321) -> (w322:errorcluster)
          }
          event "Process all errored entries": Value Change {
            w572 = T6 1 items=["Unknown"=-1, "Storage"=0, "Processing"=1, "Unmerged"=2] ("File Location")
            n204 = event-data() -> ()  [unwired: 1 in, 6 out]
            n205 = local write "Live Run?"(FALSE ("Timed out?")) -> ()
            n206 = property on="Process all errored entries" class="Bool (strict)"(error in=w582, "Value"=TRUE ("Process all errored entries"), "DisabledEnum"=T3."Disabled and Grayed Out" ("Disabled")) -> (error out=w578:errorcluster)  [unwired: 1 in, 1 out]
            n207 = local read "Small?"() -> (w583:bool)
            n208 = local write "Timed out?"(TRUE ("Timed out?")) -> ()
            n209 = Number To Decimal String(number=w572) -> (decimal integer string=w573:string)  [unwired: 1 in]
            n210 = Select(t="dust_event_small", s=w583, f="dust_event") -> (s? t:f=w571:string)
            n211 = Format Into String(format string="UPDATE\n  %s\nSET\n  file_location = ?\nWHERE\n  estimate_quality < 0;", w571) -> (resulting string=w577:string)  [unwired: 2 in, 1 out]
            n212 = Build Array(w573) -> (w574:string[])
            n213 = call <userlib>:"DB_Query.vi"("error in (no error)"=w578, "Parameters"=w574, "Parameterized Query"=w577) -> ("error out"=w576:errorcluster)  [unwired: 6 in, 2 out]
            n214 = property on="Tab Control" class="TabCtl (strict)"(error in=w576, "Value"=T1."Controls" ("Tab Control")) -> (error out=w586:errorcluster)  [unwired: 1 in, 1 out]
          }
          event "Upper Time Stamp", "Lower Time Stamp": Mouse Down {
            n215 = event-data() -> ()  [unwired: 1 in, 6 out]
            n216 = property on="Process old data" class="Bool (strict)"(error in=w588, "DisabledEnum"=T3."Disabled and Grayed Out" ("Disabled")) -> (error out=w587:errorcluster)  [unwired: 1 in, 1 out]
          }
          event "Search Times": Value Change {
            w592 = T6 0 items=["Unknown"=-1, "Storage"=0, "Processing"=1, "Unmerged"=2] ("File Location")
            n217 = event-data() -> ()  [unwired: 1 in, 6 out]
            n218 = call <userlib>:"LV_to_int_time.vi"("Time Stamp"="Lower Time Stamp") -> ("Integer Time"=w593:i64)  [unwired: 8 in, 1 out]
            n219 = call <userlib>:"LV_to_int_time.vi"("Time Stamp"="Upper Time Stamp") -> ("Integer Time"=w594:i64)  [unwired: 8 in, 1 out]
            n220 = Build Array(w594, w593, w592) -> (w591:i64[])
            n221 = local write "Timed out?"(TRUE ("Timed out?")) -> ()
            n222 = property on="Search Times" class="Bool (strict)"(error in=w604, "Value"=TRUE ("Search Times"), "DisabledEnum"=T3."Disabled" ("Disabled")) -> (error out=w598:errorcluster)  [unwired: 1 in, 1 out]
            n223 = local read "Small?"() -> (w610:bool)
            n224 = Select(t="dust_event_small" ("input 1"), s=w610, f="dust_event" ("input 1")) -> (s? t:f=w611:string)
            n225 = Number To Decimal String(number=w591) -> (decimal integer string=w590:string[])  [unwired: 1 in]
            n226 = Format Into String(format string="SELECT\n  COUNT(id_dust_event)\nFROM\n  %s\nWHERE\n  integer_timestamp <= ?\n    AND\n  integer_timestamp >= ?\n    AND\n  file_location = ?;", w611) -> (resulting string=w595:string)  [unwired: 2 in, 1 out]
            n227 = call <userlib>:"DB_Query.vi"("error in (no error)"=w598, "Parameters"=w590, "Parameterized Query"=w595) -> ("error out"=w597:errorcluster, "Results"=w596:variant[][])  [unwired: 6 in, 1 out]
            n228 = Index Array(array=w596) -> (element=w622:variant[])  [unwired: 2 in]
            n229 = Index Array(array=w622) -> (element=w623:variant)  [unwired: 1 in]
            n230 = xnode "Database Variant To Data"("database variant"=w623, "error in (no error)"=w597, "type"=0) -> ("data"=w616:i32, "error out"=w599:errorcluster)
            n231 = local read "Processing Frequency (Hz):"() -> (w617:ext)
            n232 = local write "Total Events"(w616) -> ()
            n233 = property on="Process old data" class="Bool (strict)"(error in=w599, "DisabledEnum"=T3."Enabled" ("Disabled")) -> (error out=w602:errorcluster)  [unwired: 1 in, 1 out]
            n234 = Get Date/Time In Seconds() -> (seconds since 1Jan1904=w615:timestamp)
            n235 = Divide(x=w616, y=w617) -> (x/y=w606:ext)
            n236 = property on="Search Times" class="Bool (strict)"(error in=w602, "Value"=FALSE ("Search Times"), "DisabledEnum"=T3."Enabled" ("Disabled")) -> (error out=w612:errorcluster)  [unwired: 1 in, 1 out]
            n237 = Add(x=w615, y=w606) -> (x+y=→"Estimate stop time":timestamp)
            n238 = call <userlib>:"relative_time_to_string.vi"("Seconds"=w606) -> ("String time"=→"Estimate time to process":string)
          }
          event "Process old data": Value Change {
            w661 = T6 1 items=["Unknown"=-1, "Storage"=0, "Processing"=1, "Unmerged"=2] ("File Location")
            w658 = T6 0 items=["Unknown"=-1, "Storage"=0, "Processing"=1, "Unmerged"=2] ("File Location")
            n239 = event-data() -> ()  [unwired: 1 in, 6 out]
            n240 = local read "Lower Time Stamp"() -> (w679:timestamp)
            n241 = local read "Upper Time Stamp"() -> (w680:timestamp)
            n242 = local write "Timed out?"(TRUE ("Timed out?")) -> ()
            n243 = local write "Live Run?"(FALSE ("Timed out?")) -> ()
            n244 = call <userlib>:"LV_to_int_time.vi"("Time Stamp"=w680) -> ("Integer Time"=w660:i64)  [unwired: 8 in, 1 out]
            n245 = call <userlib>:"LV_to_int_time.vi"("Time Stamp"=w679) -> ("Integer Time"=w659:i64)  [unwired: 8 in, 1 out]
            n246 = local read "Small?"() -> (w676:bool)
            n247 = Build Array(w661, w660, w659, w658) -> (w662:i64[])
            n248 = Select(t="dust_event_small" ("input 1"), s=w676, f="dust_event" ("input 1")) -> (s? t:f=w673:string)
            n249 = Number To Decimal String(number=w662) -> (decimal integer string=w657:string[])  [unwired: 1 in]
            n250 = Format Into String(format string="UPDATE\n  %s\nSET\n  file_location = ?\nWHERE\n  integer_timestamp <= ?\n    AND\n  integer_timestamp >= ?\n    AND\n  file_location = ?;", w673) -> (resulting string=w664:string)  [unwired: 2 in, 1 out]
            n251 = call <userlib>:"DB_Query.vi"("error in (no error)"=w663, "Parameters"=w657, "Parameterized Query"=w664) -> ("error out"=w665:errorcluster)  [unwired: 6 in, 2 out]
            n252 = property on="Process old data" class="Bool (strict)"(error in=w665, "DisabledEnum"=T3."Disabled and Grayed Out" ("Disabled")) -> (error out=w668:errorcluster)  [unwired: 1 in, 1 out]
            n253 = property on="Process all errored entries" class="Bool (strict)"(error in=w668, "DisabledEnum"=T3."Disabled and Grayed Out" ("Disabled")) -> (error out=w667:errorcluster)  [unwired: 1 in, 1 out]
            n254 = property on="Search Times" class="Bool (strict)"(error in=w667, "DisabledEnum"=T3."Disabled and Grayed Out" ("Disabled")) -> (error out=w666:errorcluster)  [unwired: 1 in, 1 out]
            n255 = property on="Tab Control" class="TabCtl (strict)"(error in=w666, "Value"=T1."Controls" ("Tab Control")) -> (error out=w677:errorcluster)  [unwired: 1 in, 1 out]
          }
          event "stop": Value Change {
            n256 = event-data() -> ()  [unwired: 1 in, 6 out]
          }
        }
        n257 = case shown="No Error" w266 {
          selector: w266 -> [w686 w690]
          tunnel: [w686 w691] -> w265
          tunnel: [w685 w690] -> w264
          frame No Error {
            n258 = case shown="True" "Clear IDL Errors" {
              tunnel: w686 -> [_ w689]
              tunnel: [w688 w689] -> w685
              frame False {
                n259 = local read "IDL Errors"() -> (w688:errorcluster)
              }
              frame True {
                n260 = local write "IDL Errors"(w689) -> ()
              }
            }
          }
          frame Error {
            n261 = local write "IDL Errors"(w690) -> ()
            n262 = call <vilib>:"Clear Errors.vi"("error in (no error)"=w690) -> ("error out"=w691:errorcluster)  [unwired: 6 in]
          }
        }
      }
      n263 = local read "Small?"() -> (w39:bool)
      n264 = case shown="False" w39 {
        tunnel: w40 -> [w69 w235]
        tunnel: [w68 w235] -> w36
        frame False {
          n265 = while {
            shift-right: [w75] -> w68
            shift-left: w69 -> [w78]
            stop <- w73 stop-if-true
            n266 = call <userlib>:"constants.vi"() -> ("DCS Temp filepath"=w72:path)  [unwired: 3 out]
            n267 = List Folder(path=w72, error in=w78) -> (filenames=w70:string[], error out=w77:errorcluster)  [unwired: 2 in, 2 out]
            n268 = call-poly <userlib>:"Empty Array__ogtk.vi"("Array"=w70) -> ("Empty Array?"=w71:bool)  [unwired: 8 in]
            n269 = case shown="False" w71 {
              tunnel: w77 -> [w97 w234]
              tunnel: [w86 w234] -> w75
              tunnel: w70 -> [w91 _]
              frame False {
                w88 = i64 20  # Timestamp tolerance (ms)
                # "Slices the last five characters of the string\n('.hdf5') off the end."
                n270 = Array Max & Min(array=w91) -> (min value=w89:string)  [unwired: 3 out]
                n271 = call <userlib>:"Slice String 1__ogtk.vi"("Subset (i:j)"=":-5", "String"=w89) -> ("Substring (String[i:j])"=w90:string)  [unwired: 7 in]
                n272 = Decimal String To Number(string=w90, default (0L)=i64 0 ("default (0 I32)")) -> (number=w96:i64)  [unwired: 1 in, 1 out]
                n273 = Initialize Array(w90, 2 ("dimension size")) -> (w87:string[])
                n274 = Format Into String(format string="SELECT\n  id_dust_event,\n  integer_timestamp\nFROM\n  dust_event\nWHERE\n  integer_timestamp <= ? + %1$d\n    AND\n  integer_timestamp >= ? - %1$d;" ("Parameterized Query"), w88) -> (resulting string=w94:string)  [unwired: 2 in, 1 out]
                n275 = call <userlib>:"DB_Query.vi"("error in (no error)"=w97, "Parameters"=w87, "Parameterized Query"=w94) -> ("error out"=w85:errorcluster, "Results"=w84:variant[][])  [unwired: 6 in, 1 out]
                n276 = for {
                  tunnel: w84 -> [w106] mode=indexing
                  tunnel: [w98] -> w81 mode=indexing
                  shift-right: [w102] -> _
                  shift-left: _ -> [w104]
                  tunnel: [w99] -> w80 mode=indexing
                  tunnel: [w98] -> w82
                  w100 = i64 0
                  n277 = Index Array(array=w106) -> (element #1=w105:variant, element #2=w101:variant)  [unwired: 2 in]
                  n278 = xnode "Database Variant To Data"("database variant"=w105, "error in (no error)"=w104, "type"=w100) -> ("data"=w98:i64, "error out"=w103:errorcluster)
                  n279 = xnode "Database Variant To Data"("database variant"=w101, "error in (no error)"=w103, "type"=w100) -> ("data"=w99:i64, "error out"=w102:errorcluster)
                }
                n280 = Not Equal To 0?(x=w82) -> (x != 0?=w83:bool)
                n281 = case shown="True" w83 {
                  tunnel: w85 -> [w193 w220]
                  tunnel: [w184 w213] -> w86
                  tunnel: w96 -> [w186 w215]
                  tunnel: w88 -> [w180 w211]
                  tunnel: w87 -> [_ w212]
                  tunnel: w81 -> [w179 _]
                  tunnel: w80 -> [w178 _]
                  frame True {
                    n282 = Subtract(x=w180, y=w178) -> (x-y=w182:i64[])
                    n283 = Absolute Value(x=w182) -> (abs(x)=w177:i64[])
                    n284 = call <userlib>:"constants.vi"() -> ("Processed HDF5 filepath"=w176:path, "DCS Temp filepath"=w191:path)  [unwired: 2 out]
                    n285 = Array Max & Min(array=w177) -> (min index (indices)=w181:i32)  [unwired: 3 out]
                    n286 = Index Array(array=w179, index=w181) -> (element=w175:i64)
                    n287 = Quotient & Remainder(x=w175, y=i64 1000) -> (floor(x/y)=w173:i64)  [unwired: 1 out]
                    n288 = Number To Decimal String(number=w173) -> (decimal integer string=w172:string)  [unwired: 1 in]
                    n289 = Build Path(base path=w176, name or relative path=w172) -> (appended path=w171:path)
                    n290 = Build Array(w175, w186) -> (w192:i64[])
                    n291 = Build Array(w171, w191) -> (w190:path[])
                    n292 = for {
                      tunnel: w192 -> [w208] mode=indexing
                      tunnel: w190 -> [w205] mode=indexing
                      tunnel: [w203] -> w189 mode=indexing
                      n293 = Number To Decimal String(number=w208) -> (decimal integer string=w207:string)  [unwired: 1 in]
                      n294 = Concatenate Strings(w207, ".hdf5" ("string")) -> (w204:string)
                      n295 = Build Path(base path=w205, name or relative path=w204) -> (appended path=w203:path)
                    }
                    n296 = Index Array(array=w189) -> (element #1=w188:path, element #2=w187:path)  [unwired: 2 in]
                    n297 = call <userlib>:"Merge_h5_files.vi"("error in (no error)"=w193, "File to be copied in"=w187, "Original File"=w188) -> ("error out"=w183:errorcluster)  [unwired: 8 in]
                    n298 = Unbundle By Name(w183) -> ("status"=w185:bool)
                    n299 = case shown="False" w185 {
                      tunnel: w183 -> [w201 w202]
                      tunnel: [w200 w202] -> w184
                      tunnel: w175 -> [w194 _]
                      frame False {
                        w199 = T6 1 items=["Unknown"=-1, "Storage"=0, "Processing"=1, "Unmerged"=2] ("File Location")
                        n300 = Number To Decimal String(number=w199) -> (decimal integer string=w198:string)  [unwired: 1 in]
                        n301 = Number To Decimal String(number=w194) -> (decimal integer string=w196:string)  [unwired: 1 in]
                        n302 = Build Array(w198, w196) -> (w197:string[])
                        n303 = call <userlib>:"DB_Query.vi"("error in (no error)"=w201, "Parameters"=w197, "Parameterized Query"="UPDATE\n  dust_event\nSET\n  file_location = ?\nWHERE\n  id_dust_event = ?;") -> ("error out"=w200:errorcluster)  [unwired: 6 in, 2 out]
                      }
                      frame True {
                      }
                    }
                  }
                  frame False {
                    n304 = Number To Decimal String(number=w215) -> (decimal integer string=w219:string)  [unwired: 1 in]
                    n305 = Concatenate Strings(w219, ".hdf5" ("string")) -> (w217:string)
                    n306 = call <userlib>:"constants.vi"() -> ("DCS Temp filepath"=w216:path)  [unwired: 3 out]
                    n307 = Build Path(base path=w216, name or relative path=w217) -> (appended path=w214:path)
                    n308 = Delete(path (use dialog)=w214, error in=w220) -> (error out=w209:errorcluster)  [unwired: 3 in, 2 out]
                    n309 = Unbundle By Name(w209) -> ("status"=w210:bool)
                    n310 = case shown="False" w210 {
                      tunnel: [w231 w232] -> w213
                      tunnel: w209 -> [w223 w232]
                      tunnel: w212 -> [w222 _]
                      tunnel: w211 -> [w221 _]
                      frame False {
                        w225 = T6 2 items=["Unknown"=-1, "Storage"=0, "Processing"=1, "Unmerged"=2] ("File Location")
                        w229 = T6 1 items=["Unknown"=-1, "Storage"=0, "Processing"=1, "Unmerged"=2] ("File Location")
                        n311 = Number To Decimal String(number=w229) -> (decimal integer string=w228:string)  [unwired: 1 in]
                        n312 = Number To Decimal String(number=w225) -> (decimal integer string=w224:string)  [unwired: 1 in]
                        n313 = Format Into String(format string="UPDATE\n  dust_event\nSET\n  file_location = ?\nWHERE\n  integer_timestamp <= ? + %1$d\n    AND\n  file_location = ?;" ("Parameterized Query"), w221) -> (resulting string=w226:string)  [unwired: 2 in, 1 out]
                        n314 = Build Array (concatenate)(w228, w222, w224) -> (w227:string[])
                        n315 = call <userlib>:"DB_Query.vi"("error in (no error)"=w223, "Parameters"=w227, "Parameterized Query"=w226) -> ("error out"=w231:errorcluster)  [unwired: 6 in, 2 out]
                      }
                      frame True {
                      }
                    }
                  }
                }
              }
              frame True {
                n316 = Wait (ms)(milliseconds to wait=u32 100) -> ()  [unwired: 1 out]
              }
            }
            n317 = Unbundle By Name(w75) -> ("status"=w74:bool)
            n318 = local read "stop"() -> (w76:bool)
            n319 = Or(x=w74, y=w76) -> (x .or. y?=w73:bool)
          }
        }
        frame True {
        }
      }
      n320 = Merge Errors(w38, w36) -> (w37:errorcluster)
      n321 = property on="stop" class="Bool (strict)"(error in=w65, "Value"=FALSE ("stop")) -> ()  [unwired: 1 in, 2 out]
    }
  }
  "IDL Errors" <- w14
